vi "NBFM Modulation Demo.vi"() -> ()   [LabVIEW 2013]
uses:
  <vilib>/addons/Modulation/Analog/MT Passband PLL.vi
  <vilib>/express/express analysis/Spectral/Block/exnSpectralBlock spectral measurements RMS poly.vi
  <vilib>/express/express analysis/Spectral/Block/exnSpectralBlock spectral measurements RMS DDT.vi
  <vilib>/express/express analysis/Spectral/XNode/ExpressSpectralMeasurementsBlockNode.xnode
  <vilib>/addons/Modulation/niAMT.lvlib
panel:
  out "Estimated Freq.":dbl=100000.0 caption="Frequency"
  in  "Mod. Freq.":dbl=2000.0 caption="Frequency"
  in  "WAV SR":dbl=44100.0 caption="dt"
  in  "LPF Cut-Off":dbl=5000.0 caption="Lower Cut-Off"
  in  "SNR (dB)":dbl(slide)=30.0 caption="Standard deviation" scale=-20.0..50.0
  out "Recovered Signal":dynamicdata(graph)
  out "Baseband":dynamicdata(graph)
  out "FM FFT":dynamicdata(graph)
  out "FM Wave":dynamicdata(graph)
  in  "Carrier Amp.":dbl=1.0 caption="Amplitude"
  in  "stop":bool
  in  "Frequency Deviation":dbl(slide)=200.0 scale=0.0..400.0
  in  "Carrier Freq.":dbl=100000.0 caption="Frequency"
  # "Frequency Modulation"
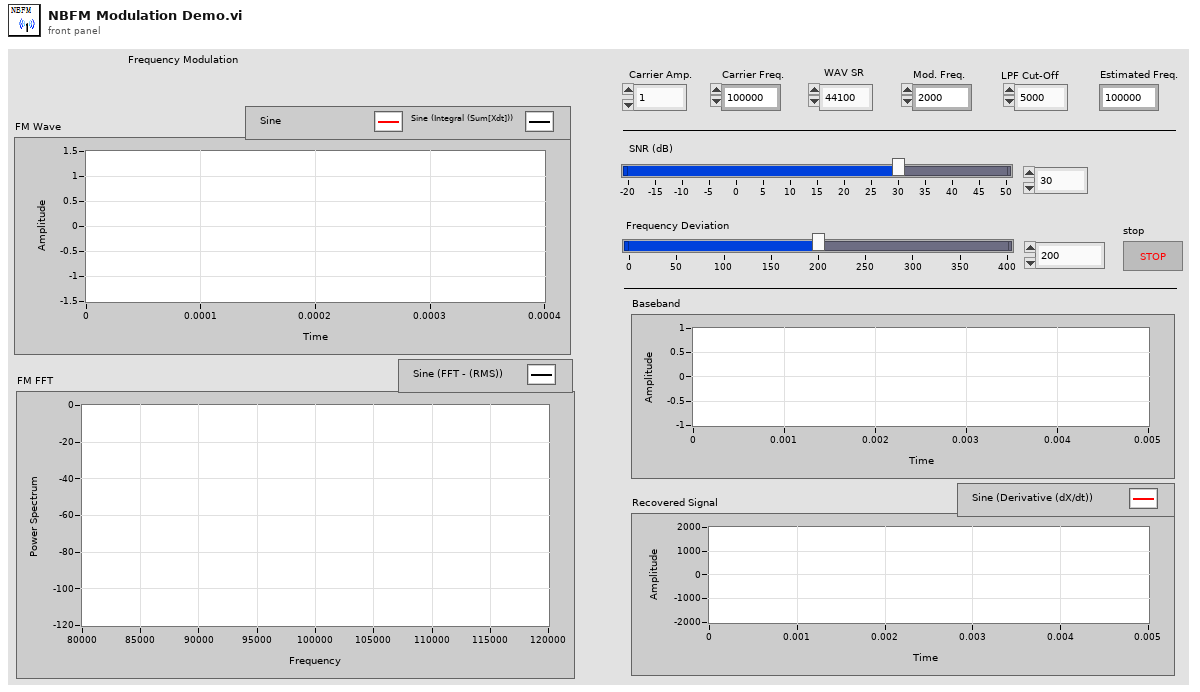
[diagram p1: front panel]
types:
  T1 = cluster{"averaging mode":u16, "weighting mode":u16, "number of averages":u32}
  T2 = cluster{"dB On (F)":bool, "unwrap phase (F)":bool, "convert to degree (F)":bool}
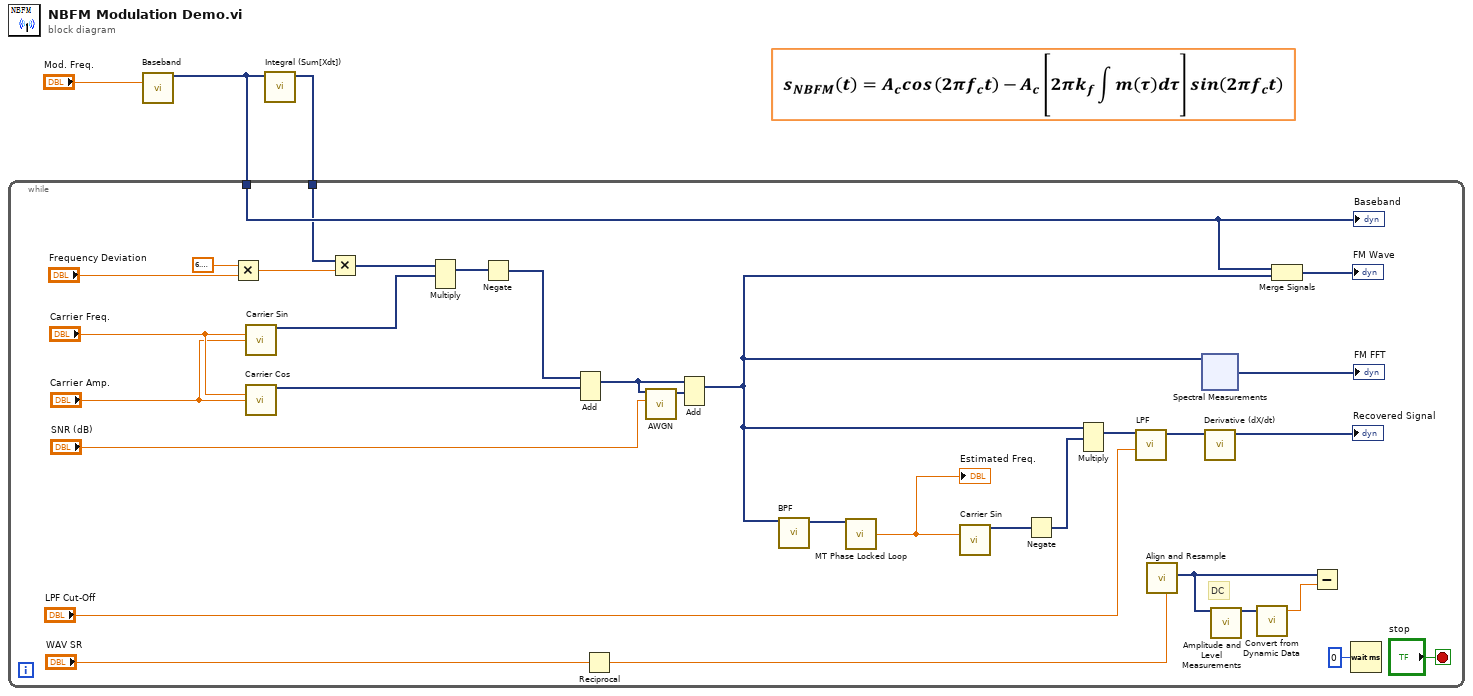
[diagram p0: block diagram]
diagram:
  n1 = call "Baseband"("Frequency"="Mod. Freq.") -> ("Sine"=w2:dynamicdata)  [unwired: 13 in, 1 out]
  n2 = call "Integral (Sum[Xdt])"("Signals"=w2) -> ("Result"=w1:dynamicdata)  [unwired: 5 in, 1 out]
  n3 = while {
    tunnel: w2 -> [w33]
    tunnel: w1 -> [w28]
    stop <- "stop" stop-if-true
    # "DC"
    n4 = Multiply(x=6.283185307179586, y="Frequency Deviation") -> (x*y=w25:dbl)
    n5 = call "Carrier Sin"("Frequency"="Carrier Freq.", "Amplitude"="Carrier Amp.") -> ("Sine"=w21:dynamicdata)  [unwired: 12 in, 1 out]
    n6 = call "Carrier Cos"("Frequency"="Carrier Freq.", "Amplitude"="Carrier Amp.") -> ("Sine"=w18:dynamicdata)  [unwired: 12 in, 1 out]
    n7 = Multiply(x=w28, y=w25) -> (x*y=w24:dynamicdata)
    n8 = Multiply(1:w21, 2:w24) -> (0:w20:dynamicdata)  [unwired: 1 in, 1 out]
    n9 = Negate(x=w20) -> (-x=w19:dynamicdata)
    n10 = Add(1:w18, 2:w19) -> (0:w16:dynamicdata)  [unwired: 1 in, 1 out]
    n11 = Reciprocal(x="WAV SR") -> (1/x=w5:dbl)
    n12 = call "AWGN.vi"("SNR (dB)"="SNR (dB)", "Dynamic Data"=w16) -> ("DC with Gaussian Noise"=w17:dynamicdata)  [unwired: 9 in]
    n13 = Add(1:w17, 2:w16) -> (0:w10:dynamicdata)  [unwired: 1 in, 1 out]
    n14 = call "BPF"("Signal"=w10) -> ("Filtered Signal"=w6:dynamicdata)  [unwired: 9 in, 1 out]
    n15 = call-poly <vilib>:"MT Phase Locked Loop.vi"("passband waveform"=w6) -> ("estimated carrier frequency (Hz)"=w12:dbl)  [unwired: 10 in, 4 out]
    "Estimated Freq." <- w12
    n16 = call "Carrier Sin"("Frequency"=w12) -> ("Sine"=w13:dynamicdata)  [unwired: 13 in, 1 out]
    n17 = Negate(x=w13) -> (-x=w7:dynamicdata)
    n18 = Multiply(1:w7, 2:w10) -> (0:w11:dynamicdata)  [unwired: 1 in, 1 out]
    n19 = call "LPF"("Lower Cut-Off"="LPF Cut-Off", "Signal"=w11) -> ("Filtered Signal"=w9:dynamicdata)  [unwired: 8 in, 1 out]
    n20 = call "Align and Resample"("dt"=w5) -> ("Resampled Signals"=w31:dynamicdata)  [unwired: 8 in, 2 out]
    n21 = xnode ("Spectral Measurements")("Signals"=w10) -> ("FFT - (RMS)"=→"FM FFT":dynamicdata)  [unwired: 1 in, 2 out]
    n22 = call "Derivative (dX/dt)"("Signals"=w9) -> ("Result"=→"Recovered Signal":dynamicdata)  [unwired: 5 in, 1 out]
    n23 = call "Amplitude and Level Measurements"("Signals"=w31) -> ("Mean (DC)"=w30:dynamicdata)  [unwired: 13 in, 1 out]
    n24 = call "Convert from Dynamic Data"("Dynamic Data Type"=w30) -> ("Scalar"=w32:dbl)  [unwired: 3 in]
    n25 = Merge Signals(w33, w10) -> (→"FM Wave":dynamicdata)
    n26 = Subtract(x=w31, y=w32) -> ()  [unwired: 1 out]
    n27 = Wait (ms)(milliseconds to wait=u32 0) -> ()  [unwired: 1 out]
    "Baseband" <- w33
  }
